vi "test_Set FPGA Bitfile_Error.vi"(8 "error in (no error)":errorcluster, 11 "TestCase in":refnum<class "FPGA Addon Scripting API Unit Tests.lvclass">=refnum) -> (0 "error out":errorcluster, 3 "TestCase out":refnum<class "FPGA Addon Scripting API Unit Tests.lvclass">)   [LabVIEW 2026, in "FPGA Addon Scripting API Unit Tests.lvclass"]
uses:
  FPGA Addon Scripting API Unit Tests.lvclass
  FPGA Addon Test Class/FPGA Addon Test Class.lvclass
  APIs/Scripting API/Scripting API.lvlib
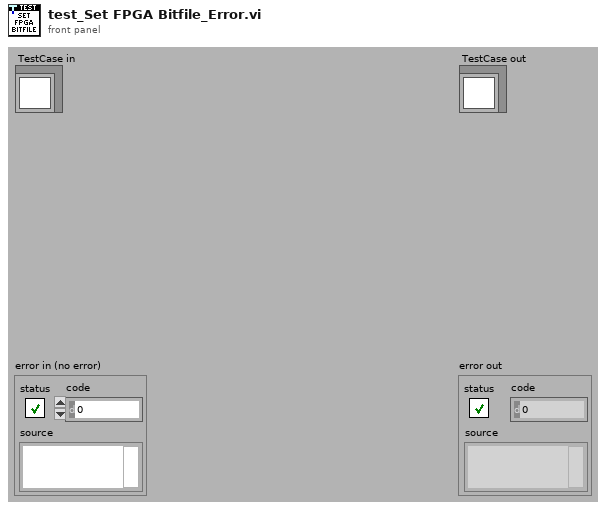
[diagram p1: front panel]
types:
  T1 = typedef "Custom Device API.lvlib/Custom Device Item Ref.ctl" = u64
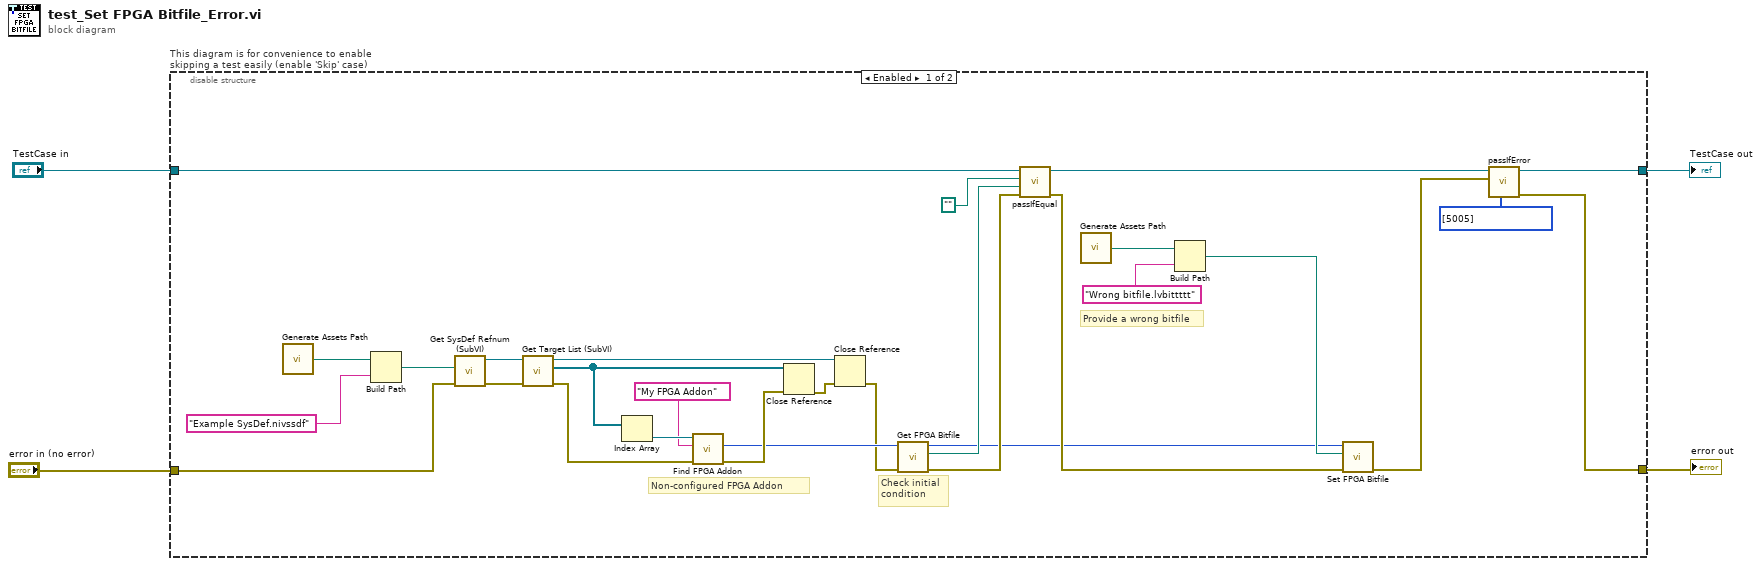
[diagram p0: block diagram]
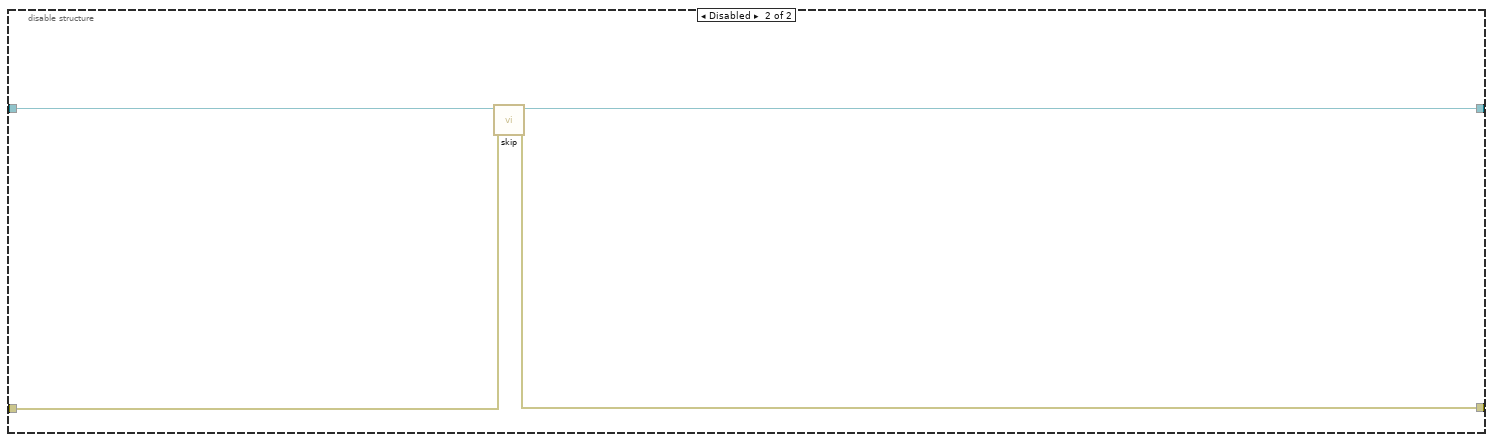
[diagram p2: hidden frame]
diagram:
  n1 = disable-structure "This diagram is for convenience to enable skipping a test easily (enable 'Skip' case)" shown="Enabled" {
    disable-tunnel: "TestCase in" -> [w15 w37]
    disable-tunnel: [w8 w35] -> w1
    disable-tunnel: [w5 w36] -> w3
    disable-tunnel: "error in (no error)" -> [w29 w34]
    frame Enabled {
      # "Provide a wrong bitfile"
      # "Check initial condition"
      # "Non-configured FPGA Addon"
      n2 = call "Generate Assets Path.vi"() -> ("Assets path"=w33:path)
      n3 = Build Path(base path=w33, name or relative path="Example SysDef.nivssdf") -> (appended path=w31:path)
      n4 = call "Get SysDef Refnum (SubVI).vi"("error in (no error)"=w29, "System Definition path"=w31) -> ("error out"=w28:errorcluster, "NationalInstruments.VeriStand.SystemDefinitionAPI.SystemDefinition"=w30:refnum<k39>)  [unwired: 8 in]
      n5 = call "Get Target List (SubVI).vi"("error in (no error)"=w28, "NationalInstruments.VeriStand.SystemDefinitionAPI.SystemDefinition"=w30) -> ("error out"=w23:errorcluster, "Target List Refnums"=w27:refnum<k39>[], "NationalInstruments.VeriStand.SystemDefinitionAPI.SystemDefinition"=w26:refnum<k39>)  [unwired: 7 in]
      n6 = Index Array(array=w27) -> (element=w24:refnum<k39>)  [unwired: 1 in]
      n7 = call "Find FPGA Addon.vi"("error in"=w23, "FPGA addon name"="My FPGA Addon", "NationalInstruments.VeriStand.SystemDefinitionAPI.Target"=w24) -> ("error out"=w21:errorcluster, "FPGA addon refnum out"=w17:T1)  [unwired: 5 in, 2 out]
      n8 = Close Reference(reference=w27, error in (no error)=w21) -> (error out=w25:errorcluster)
      n9 = Close Reference(reference=w26, error in (no error)=w25) -> (error out=w16:errorcluster)
      n10 = call "Get FPGA Bitfile.vi"("error in"=w16, "FPGA addon refnum in"=w17) -> ("error out"=w13:errorcluster, "FPGA bitfile path"=w14:path, "FPGA addon refnum out"=w10:T1)  [unwired: 7 in]
      n11 = call-dynamic "passIfEqual.vi"("error in (no error)"=w13, "y"=w14, "x"=path "", "TestCase in"=w15) -> ("error out"=w12:errorcluster, "TestCase out"=w9:refnum<class "FPGA Addon Scripting API Unit Tests.lvclass">)  [unwired: 6 in]
      n12 = call "Generate Assets Path.vi"() -> ("Assets path"=w20:path)
      n13 = Build Path(base path=w20, name or relative path="Wrong bitfile.lvbittttt") -> (appended path=w18:path)
      n14 = call "Set FPGA Bitfile.vi"("error in"=w12, "FPGA bitfile path"=w18, "FPGA addon refnum in"=w10) -> ("error out"=w7:errorcluster)  [unwired: 7 in, 1 out]
      n15 = call-dynamic "passIfError.vi"("passing error codes (default = any error code)"=i32[] [5005], "error"=w7, "TestCase in"=w9) -> ("error out"=w5:errorcluster, "TestCase out"=w8:refnum<class "FPGA Addon Scripting API Unit Tests.lvclass">)  [unwired: 7 in]
    }
    frame Disabled {
      # "skip test result while test is under development"
      n16 = call <vilib>:"skip.vi"("error in (no error)"=w34, "TestCase in"=w37) -> ("error out"=w36:errorcluster, "TestCase out"=w35:refnum<class "FPGA Addon Scripting API Unit Tests.lvclass">)  [unwired: 8 in]
    }
  }
  "error out" <- w3
  "TestCase out" <- w1
